vi "PH_Img_BaseClass.constructor.vi"(0 "name":string, 2 "data in":string, 5 "error in(no error)":errorcluster) -> (14 "i ref out":refnum<vi>, 16 "data out":string, 19 "error out":errorcluster)   [LabVIEW 2014, in "PH_Img_BaseClass.lvlib"]
doc: "This is the constructor of a class.\n\nLicense Agreement for this software:\n\nCopyright (C)\nGesellschaft für Schwerionenforschung, GSI\nPlanckstr. 1\n64291 Darmstadt\nGermany\n\nContact: D.Beck@gsi.de \n\nThis program is free software; you can redistribute it and/or modify it under the terms of the \nGNU General Public License as published by the Free Software Foundation; either version 2 of \nthe license, or (at your option) any later version.\n\nThis program is distributed in the hope that it will be useful, but WITHOUT ANY WARRANTY; \nwithout even the implied warranty of MERCHANTABILITY or FITNESS FOR A PARTICULAR PURPOSE. See the GNU General License for more details (http://www.gnu.org).\n\nGesellschaft für Schwerionenforschung, GSI\nPlanckstr. 1, 64291 Darmstadt, Germany\nFor all questions and ideas contact: M.Richter@gsi.de, H.Brand@gsi.de or D.Beck@gsi.de.\nLast update: 16-JUN-2004"
uses:
  PH_Img_BaseClass.lvlib
  PH_Img_BaseClass.i attribute.ctl
  PH_Img_BaseClass.GUI Refs.ctl
  PH_Img_BaseClass.Palette.ctl
  CS_Core/CSSystem/CSSystemLib/CSSystemLib.lvlib
  PH_Class/PH_Class.lvlib
  CS_Core/BaseProcess/BaseProcess.lvlib
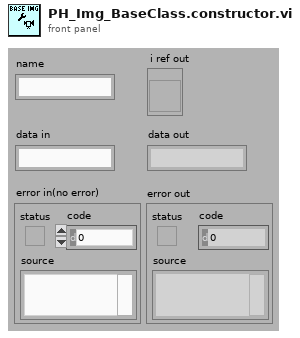
[diagram p1: front panel]
types:
  T1 = typedef "PH_Img_BaseClass.lvlib/PH_Img_BaseClass.i attribute.ctl" = cluster{"GUI Refs":T2, "Timeout Image [ms]":i32, "Default Periodic Period [ms]":i32, "Camera":cluster{"Instancename":string, "Notifier":refnum<notifier>}, "Palette":T3, "Cam Settings":cluster{"Cam ID":string, "Gain":dbl, "Brightness":dbl, "Shutter":dbl, "Cam Info Failure":bool, "Mode":i32}}
  T2 = typedef "PH_Img_BaseClass.lvlib/PH_Img_BaseClass.GUI Refs.ctl" = cluster{"Timeout":refnum<vi>, "Image":refnum<vi>, "Palette":refnum<vi>, "Timeout Set":refnum<vi>}
  T3 = typedef "PH_Img_BaseClass.lvlib/PH_Img_BaseClass.Palette.ctl" = i32
  T4 = enum16{"SetAttribute", "GetAttribute", "CreateAttribute", "DestroyAttribute", "DestroyAllAtributes"}
  T5 = typedef "BaseProcess.lvlib/BaseProcess.i attribute.ctl" = cluster{"EventStatus":string, "EventError":i32, "PresetEvtWatchD":i32, "PresetPdcWatchD":i32, "EventTimeout":i32, "PeriodicInterval":i32, "Interface":string[], "Address":string[], "Special":string[], "PeriodicError":i32, "PeriodicStatus":string, "SuperProc":string, "Descriptors":T6[], "CaseRef":refnum<vi>, "PdcRef":refnum<vi>, "Thread Ref":refnum<vi>, "eventErrorID":i32, "eventStatusID":i32, "periodicErrorID":i32, "periodicStatusID":i32, "pdcCtrID":i32}
  T6 = typedef "BaseProcess.lvlib/BaseProcess.descriptor definition.ctl" = cluster{"selector":string, "descriptor":T7}
  T7 = typedef "BaseProcess.lvlib/BaseProcess.descriptor string definition.ctl" = string
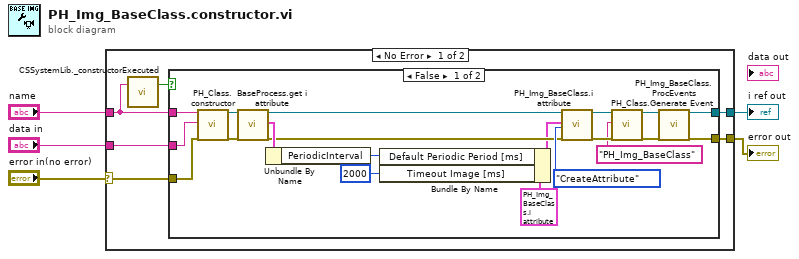
[diagram p0: block diagram]
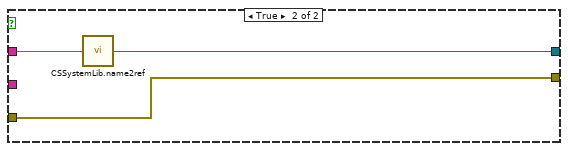
[diagram p2: hidden frame]
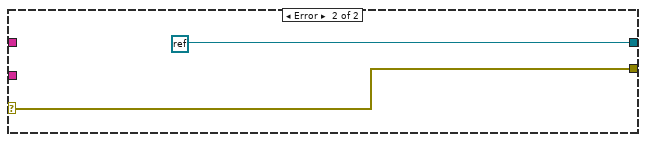
[diagram p3: hidden frame]
diagram:
  n1 = case shown="No Error" "error in(no error)" {
    selector: "error in(no error)" -> [w11 w35]
    tunnel: "name" -> [w8 _]
    tunnel: [w10 refnum<k0> refnum] -> w4
    tunnel: [w9 w35] -> w3
    tunnel: "data in" -> [w6 _]
    frame No Error {
      n2 = call "CSSystemLib._constructorExecuted.vi"("name"=w8) -> ("constructor executed?"=w7:bool)  [unwired: 18 in]
      n3 = case shown="False" w7 {
        tunnel: w11 -> [w13 w34]
        tunnel: w8 -> [w31 w33]
        tunnel: [w22 w32] -> w10
        tunnel: [w21 w34] -> w9
        tunnel: w6 -> [w12 _]
        frame False {
          n4 = call "PH_Class.constructor.vi"("name"=w31, "data in"=w12, "error in"=w13) -> ("i ref out"=w15:refnum<vi>, "error out"=w14:errorcluster)  [unwired: 14 in, 1 out]
          n5 = call "BaseProcess.get i attribute.vi"("i ref in"=w15, "error in (no error)"=w14) -> ("i ref out"=w26:refnum<vi>, "i attribute"=w30:T5, "error out"=w25:errorcluster)  [unwired: 15 in]
          n6 = Unbundle By Name(w30) -> ("PeriodicInterval"=w27:i32)
          n7 = Bundle By Name(cluster=T1 {"GUI Refs"={"Timeout"=refnum, "Image"=refnum, "Palette"=refnum, "Timeout Set"=refnum}, "Timeout Image [ms]"=1000, "Default Periodic Period [ms]"=0, "Camera"={"Instancename"="", "Notifier"=refnum}, "Palette"=0, "Cam Settings"={"Cam ID"="", "Gain"=0.0, "Brightness"=0.0, "Shutter"=0.0, "Cam Info Failure"=FALSE, "Mode"=0}} ("CLASS.i attribute"), "Default Periodic Period [ms]"=w27, "Timeout Image [ms]"=2000) -> (w23:T1)
          n8 = call "PH_Img_BaseClass.i attribute.vi"("VI Refnum"=w26, "CLASS.i attribute"=w23, "Action"=T4."CreateAttribute", "error in (no error)"=w25) -> ("VI Refnum out"=w20:refnum<vi>, "error out"=w17:errorcluster)  [unwired: 13 in, 1 out]
          n9 = call "PH_Class.Generate Event.vi"("i ref in"=w20, "Class"="PH_Img_BaseClass", "error in (no error)"=w17) -> ("i ref out"=w19:refnum<vi>, "error out"=w18:errorcluster)  [unwired: 15 in]
          n10 = call "PH_Img_BaseClass.ProcEvents.vi"("i ref in"=w19, "error in"=w18) -> ("i ref out"=w22:refnum<vi>, "error out"=w21:errorcluster)  [unwired: 16 in]
        }
        frame True {
          n11 = call "CSSystemLib.name2ref.vi"("name"=w33) -> ("obj refnum"=w32:refnum<vi>)
        }
      }
    }
    frame Error {
    }
  }
  "i ref out" <- w4
  "error out" <- w3
